vi "initialize.vi"(7 "references":T1, 8 "error in (no error)":errorcluster) -> (0 "error out":errorcluster)   [LabVIEW 2015, in "example_01.lvlib"]
uses:
  example_01.lvlib
  lv-recipe-machine/public/_controls/references.ctl
  lv-recipe-machine/public/_controls/input.ctl
  lv-recipe-machine/public/_controls/input_command.ctl
  lv-recipe-machine/public/_controls/output.ctl
  lv-recipe-machine/public/_controls/transition.ctl
  lv-recipe-machine/public/_controls/data.ctl
  lv-recipe-machine/public/_controls/configuration.ctl
  lv-recipe-machine/public/_controls/recipe_data.ctl
  lv-recipe-machine/public/_controls/mode.ctl
  lv-recipe-machine/public/_controls/manual_state.ctl
  lv-recipe-machine/public/_controls/automatic_state.ctl
  lv-recipe-machine/public/_controls/timer.ctl
  lv-recipe-machine/public/_controls/recipe_step.ctl
  lv-recipe-machine/public/_controls/change.ctl
  lv-recipe-machine/public/_controls/status.ctl
  lv-recipe-machine/lv-recipe-machine.lvlib
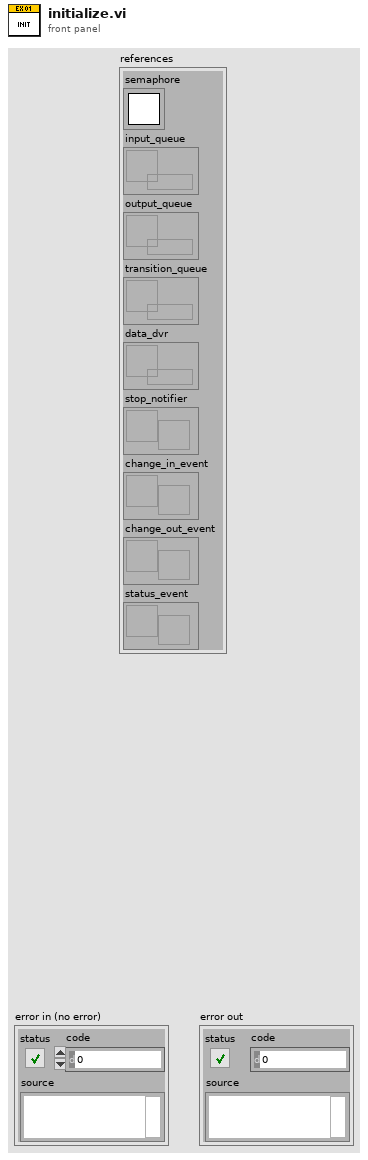
[diagram p1: front panel]
types:
  T1 = typedef "lv-recipe-machine.lvlib/references.ctl" = cluster{"semaphore":T2, "input_queue":refnum<queue>, "output_queue":refnum<queue>, "transition_queue":refnum<queue>, "data_dvr":refnum<data-value>, "stop_notifier":refnum<notifier>, "change_in_event":refnum<user-event>, "change_out_event":refnum<user-event>, "status_event":refnum<user-event>}
  T2 = typedef "Semaphore RefNum" = refnum<k1>
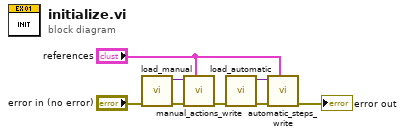
[diagram p0: block diagram]
diagram:
  n1 = call "load_manual.vi"("error in (no error)"="error in (no error)") -> ("error out"=w7:errorcluster, "manual_actions out"=w3:variant)  [unwired: 8 in, 1 out]
  n2 = call "manual_actions_write.vi"("references"="references", "error in (no error)"=w7, "manual_actions"=w3) -> ("error out"=w6:errorcluster)  [unwired: 8 in]
  n3 = call "load_automatic.vi"("error in (no error)"=w6) -> ("error out"=w5:errorcluster, "automatic_steps out"=w4:variant)  [unwired: 8 in, 1 out]
  n4 = call "automatic_steps_write.vi"("references"="references", "error in (no error)"=w5, "automatic_steps"=w4) -> ("error out"=→"error out":errorcluster)  [unwired: 7 in, 1 out]
